vi "PH_BeamlineController.set Target Elements to be enabled.vi"(0 "VI in":refnum<vi>, 5 "error in (no error)":errorcluster) -> (14 "VI out":refnum<vi>, 19 "error out":errorcluster)   [LabVIEW 2014, in "PH_BeamlineController.lvlib"]
uses:
  PH_BeamlineController.lvlib
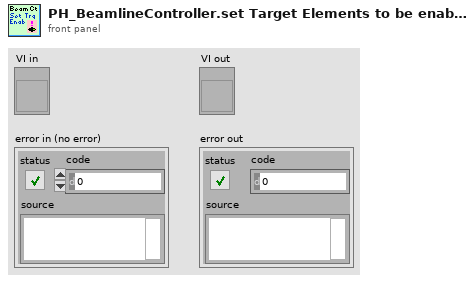
[diagram p1: front panel]
types:
  T1 = typedef "PH_BeamlineController.lvlib/PH_BeamlineController.i attribute.ctl" = cluster{"Vacuum Exp LB":cluster{"Channel":string, "Limit [mbar]":dbl, "Pressure [mbar]":dbl, "GUI Ref":refnum<vi>}, "Sources":T2[], "PA DP Targets":T4[], "Path":cluster{"Source":T3, "PA DP Target":T5, "Target":T6}, "Targets":cluster{"Name":T6, "GUI Ref":refnum<vi>, "Current State":bool, "Wanted State":bool, "Enabled":bool}[], "Status Tags":cluster{"Name":string, "Status":T7}[], "special GUI Refs":T8}
  T2 = typedef "PH_BeamlineController.lvlib/PH_BeamlineController.Source Attributes.ctl" = cluster{"Name":T3, "GUI Ref":refnum<vi>, "Current State":bool, "Wanted State":bool}
  T3 = typedef "PH_BeamlineController.lvlib/PH_BeamlineController.Sources.ctl" = enum16{"None", "YLF", "fs-Frontend", "ns-Frontend", "YLF and ns-Frontend", "fs- and ns-Frontend"}
  T4 = typedef "PH_BeamlineController.lvlib/PH_BeamlineController.PA DP Target Attributes.ctl" = cluster{"Name":T5, "GUI Ref":refnum<vi>, "Current State":bool, "Wanted State":bool, "Enabled":bool}
  T5 = typedef "PH_BeamlineController.lvlib/PH_BeamlineController.PA DP Targets.ctl" = enum16{"None", "Dump PA Delayed Beam", "Dump PA Undelayed Beam", "Dumps PA Delayed and Undelayed Beam"}
  T6 = typedef "PH_BeamlineController.lvlib/PH_BeamlineController.Targets.ctl" = enum16{"None", "PreAmp", "Dump Exp Laserlab", "Exp Laserlab", "Calorimeter", "Dump Exp Laserbay", "Exp Laserbay", "Dump Exp Z6", "Exp Z6"}
  T7 = typedef "PH_StatusHandler.lvlib/PH_StatusHandler.Status.ctl" = i16
  T8 = typedef "PH_BeamlineController.lvlib/PH_BeamlineController.special GUI Refs.ctl" = cluster{"PA-Backreflection-Meas":refnum<vi>, "fs_Synchrolock_Watch":refnum<vi>}
  T9 = cluster{"Name":T6, "GUI Ref":refnum<vi>, "Current State":bool, "Wanted State":bool, "Enabled":bool}[]
  T10 = typedef "PH_BeamlineController.lvlib/PH_BeamlineController.Target Attributes.ctl" = cluster{"Name":T6, "GUI Ref":refnum<vi>, "Current State":bool, "Wanted State":bool, "Enabled":bool}
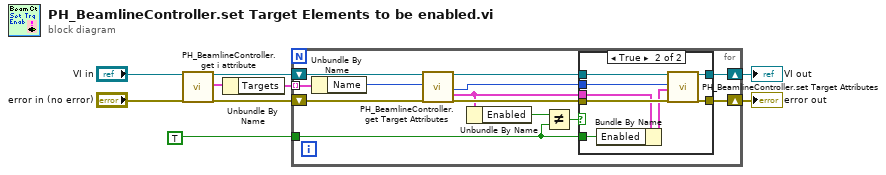
[diagram p0: block diagram]
diagram:
  n1 = call "PH_BeamlineController.get i attribute.vi"("i ref in"="VI in", "error in (no error)"="error in (no error)") -> ("i ref out"=w7:refnum<vi>, "i attribute"=w8:T1, "error out"=w9:errorcluster)  [unwired: 15 in]
  n2 = Unbundle By Name(w8) -> ("Targets"=w4:T9)
  n3 = for {
    shift-right: [w19] -> w6
    shift-left: w9 -> [w22]
    shift-right: [w17] -> w5
    shift-left: w7 -> [w20]
    tunnel: w4 -> [w15] mode=indexing
    tunnel: TRUE -> [w10]
    n4 = Unbundle By Name(w15) -> ("Name"=w11:T6)
    n5 = call "PH_BeamlineController.get Target Attributes.vi"("VI in"=w20, "Target"=w11, "error in (no error)"=w22) -> ("VI out"=w18:refnum<vi>, "Target Index"=w16:i32, "Target Attributes"=w14:T10, "error out"=w21:errorcluster)  [unwired: 13 in]
    n6 = Unbundle By Name(w14) -> ("Enabled"=w13:bool)
    n7 = Not Equal?(x=w13, y=w10) -> (x != y?=w12:bool)
    n8 = case shown="True" w12 {
      tunnel: w21 -> [w23 w32]
      tunnel: [w23 w31] -> w19
      tunnel: w18 -> [w24 w30]
      tunnel: [w24 w29] -> w17
      tunnel: w16 -> [_ w28]
      tunnel: w14 -> [_ w26]
      tunnel: w10 -> [_ w25]
      frame False {
      }
      frame True {
        n9 = Bundle By Name(cluster=w26, "Enabled"=w25) -> (w27:T10)
        n10 = call "PH_BeamlineController.set Target Attributes.vi"("VI in"=w30, "Target Index"=w28, "Changed Target Attributes"=w27, "error in (no error)"=w32) -> ("VI out"=w29:refnum<vi>, "error out"=w31:errorcluster)  [unwired: 14 in]
      }
    }
  }
  "VI out" <- w5
  "error out" <- w6
